vi "Write Owner.vi"(8 "error in (no error)":errorcluster, 10 "Owner":string, 11 "Subscription in":refnum<class "Subscription.lvclass">) -> (0 "error out":errorcluster, 3 "Subscription out":refnum<class "Subscription.lvclass">)   [LabVIEW 2015, in "NI_AWS_SNS.lvlib" / "Subscription.lvclass"]
uses:
  Subscription.lvclass
  Subscription.lvclass/Subscription.ctl
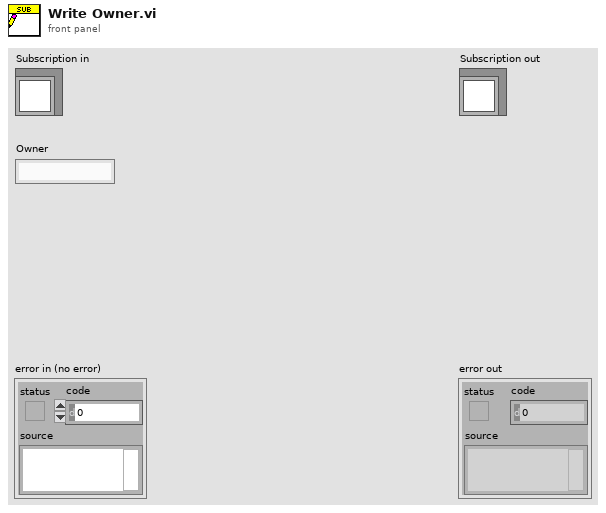
[diagram p1: front panel]
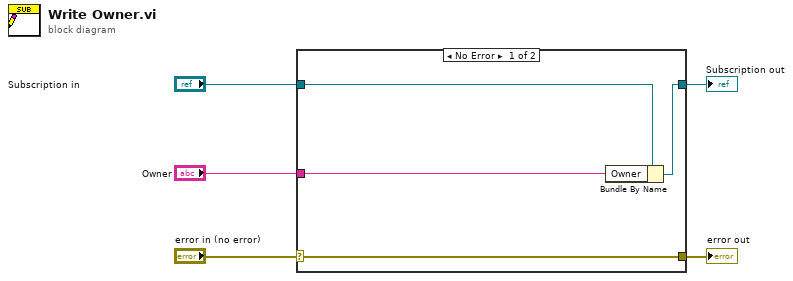
[diagram p0: block diagram]
diagram:
  n1 = case shown="No Error" "error in (no error)" {
    selector: "error in (no error)" -> [w9 w10]
    tunnel: [w9 w10] -> w4
    tunnel: [w7 w11] -> w2
    tunnel: "Subscription in" -> [w8 w11]
    tunnel: "Owner" -> [w6 _]
    frame No Error {
      n2 = Bundle By Name(cluster=w8, "Owner"=w6) -> (w7:refnum<class "Subscription.lvclass">)
    }
    frame Error {
    }
  }
  "error out" <- w4
  "Subscription out" <- w2
